vi "test_add_elements.vi"() -> ()   [LabVIEW 2018]
uses:
  add_element(array).vi
  add_element(variant).vi
panel:
  out "elapsed time in millisec (variant)":dbl
  out "elapsed time in millisec (array)":dbl
  in  "number of elements":i32=10000
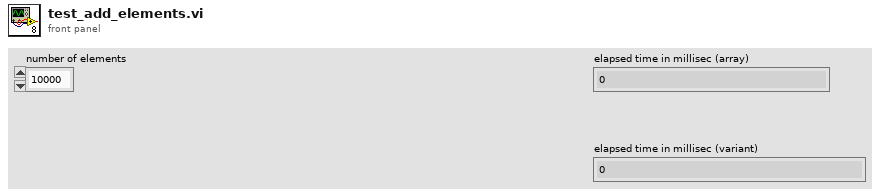
[diagram p1: front panel]
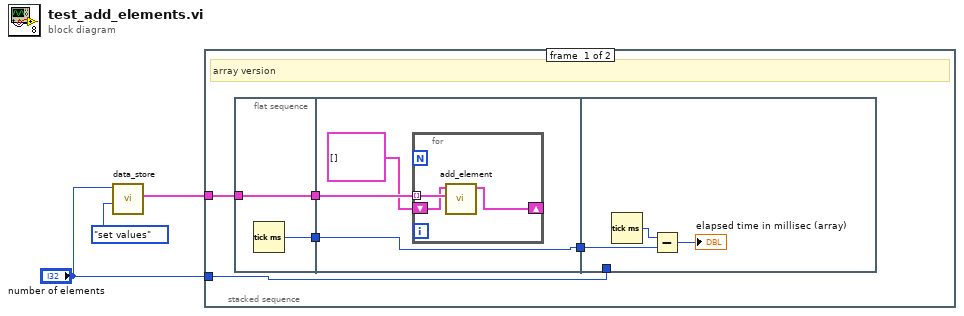
[diagram p0: block diagram]
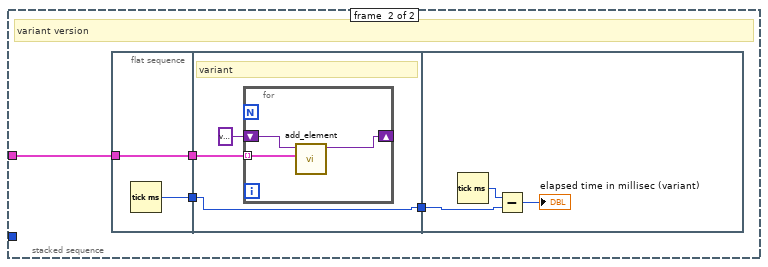
[diagram p2: hidden frame]
diagram:
  n1 = call "data_store.vi"("Action"=enum16{"set values", "get values"}."set values", "number of elements"="number of elements") -> ("array items"=w2:cluster{"name":string, "address":string}[])  [unwired: 7 in, 2 out]
  n2 = stacked-sequence {
    tunnel: "number of elements" -> [w5 _]
    tunnel: w2 -> [w4 w20]
    frame #0 {
      # "array version"
      n3 = flat-sequence {
        tunnel: [w10] -> w8
        tunnel: w4 -> [w9]
        tunnel: [w9] -> w7
        tunnel: [w13] -> w6
        tunnel: w8 -> [w13]
        tunnel: w7 -> [w12]
        tunnel: w6 -> [w18]
        tunnel: w5 -> [_]
        frame #0 {
          n4 = Tick Count (ms)() -> (millisecond timer value=w10:u32)
        }
        frame #1 {
          n5 = for {
            tunnel: w12 -> [w16] mode=indexing
            shift-right: [w15] -> _
            shift-left: cluster{"name":string, "address":string}[] [] ("data store (out)") -> [w14]
            n6 = call-poly "add_element.vi"("element"=w16, "data store (in)"=w14) -> ("data store (out)"=w15:cluster{"name":string, "address":string}[])  [unwired: 8 in, 1 out]
          }
        }
        frame #2 {
          n7 = Tick Count (ms)() -> (millisecond timer value=w19:u32)
          n8 = Subtract(x=w19, y=w18) -> (x-y=→"elapsed time in millisec (array)":u32)
        }
      }
    }
    frame #1 {
      # "variant version"
      n9 = flat-sequence {
        tunnel: [w25] -> w23
        tunnel: w20 -> [w24]
        tunnel: [w24] -> w22
        tunnel: [w28] -> w21
        tunnel: w23 -> [w28]
        tunnel: w22 -> [w27]
        tunnel: w21 -> [w33]
        frame #0 {
          n10 = Tick Count (ms)() -> (millisecond timer value=w25:u32)
        }
        frame #1 {
          # "variant"
          n11 = for {
            tunnel: w27 -> [w31] mode=indexing
            shift-right: [w29] -> _
            shift-left: variant ("data store (variant)") -> [w30]
            n12 = call-poly "add_element.vi"("element"=w31, "data store (variant)"=w30) -> ("data store (variant)"=w29:variant)  [unwired: 8 in, 1 out]
          }
        }
        frame #2 {
          n13 = Tick Count (ms)() -> (millisecond timer value=w34:u32)
          n14 = Subtract(x=w34, y=w33) -> (x-y=→"elapsed time in millisec (variant)":u32)
        }
      }
    }
  }
